vi "fgv_reg_q.vi"(7 "cmd":T2, 8 "error in":errorcluster, 11 "action":T1) -> (0 "error out":errorcluster, 3 "queue out":refnum<queue>)   [LabVIEW 2019]
uses:
  _ctrl/create-rw-close.ctl
  q-action_reg.ctl
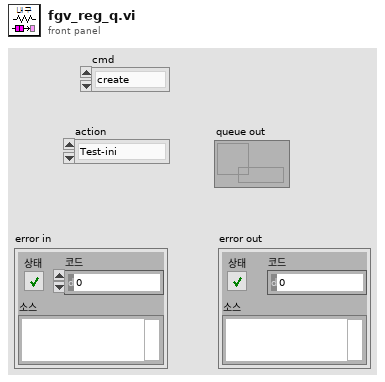
[diagram p1: front panel]
types:
  T1 = typedef "q-action_reg.ctl" = enum16{"Test-ini", "BP4610-on", "Pause", "Test-start", "Group-ini", "Ch-select", "Relay-on", "DSP-on", "DL950-start", "AO-start", "AO-delay", "Delay", "DL950-stop", "DSP-off", "Relay-off", "Ch-check", "UI-update", "Group-end", "Test-stop", "BP4610-off", "Test-finish", "Test-Manual", "DL950-Manual"}
  T2 = typedef "create-rw-close.ctl" = enum16{"create", "write", "read", "delete", "close"}
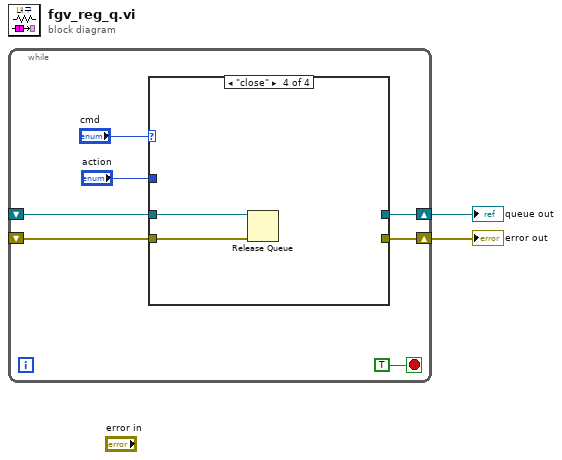
[diagram p0: block diagram]
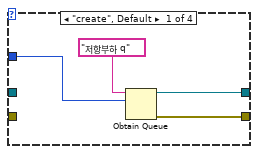
[diagram p2: hidden frame]
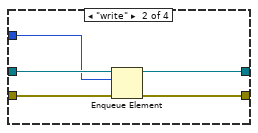
[diagram p3: hidden frame]
diagram:
  n1 = while {
    shift-right: [w7] -> w1
    shift-left: _ -> [w5]
    shift-right: [w6] -> w2
    shift-left: _ -> [w4]
    stop <- TRUE stop-if-true
    n2 = case shown="\"close\"" "cmd" {
      tunnel: [w13 w18 w20 _] -> w7
      tunnel: [w12 w17 w19 _] -> w6
      tunnel: "action" -> [w10 w14 _ _]
      tunnel: w5 -> [_ w16 w20 w21]
      tunnel: w4 -> [_ w15 w19 w22]
      frame "create", Default {
        n3 = Obtain Queue(name (unnamed)="저항부하 q" ("이름(이름없음)"), element data type=w10) -> (queue out=w13:refnum<queue>, error out=w12:errorcluster)  [unwired: 3 in, 1 out]
      }
      frame "write" {
        n4 = Enqueue Element(queue=w16, element=w14, error in (no error)=w15) -> (queue out=w18:refnum<queue>, error out=w17:errorcluster)  [unwired: 1 in, 1 out]
      }
      frame "read" {
      }
      frame "close" {
        n5 = Release Queue(queue=w21, error in (no error)=w22) -> ()  [unwired: 1 in, 3 out]
      }
    }
  }
  "error out" <- w2
  "queue out" <- w1
